vi "Begin.vi"(8 "error in":errorcluster) -> (0 "error out":errorcluster)   [LabVIEW 2020]
doc: "Called before other user functions, this VI is expected to open initial I/O refnums, load in file data, and do all program initialization. Notice that the <B>error out</B> terminal is simply used for data flow. Wiring it to other structures or subVIs ensures that this VI runs first."
uses:
  <vilib>/Rock Robotics/WPI/DriverStation/WPI_DriverStationRobotMode2.ctl
  <vilib>/Rock Robotics/WPI/ThirdParty/Phoenix-LabVIEW/Motor Controller/Controls/CTRE_Phoenix_MotorControl_FeedbackDevice_TalonFX.ctl
  <vilib>/Rock Robotics/WPI/ThirdParty/Phoenix-LabVIEW/Motor Controller/Controls/CTRE_Phoenix_MotorControl_SupplyCurrentLimitConfiguration.ctl
  <vilib>/Rock Robotics/WPI/ThirdParty/Phoenix-LabVIEW/Motor Controller/Controls/CTRE_Phoenix_MotorControl_ControlMode.ctl
  <vilib>/Rock Robotics/WPI/ThirdParty/Phoenix-LabVIEW/Motor Controller/Controls/CTRE_Phoenix_MotorControl_NeutralMode.ctl
  <vilib>/Rock Robotics/WPI/Joystick/WPI_JoystickDeviceEnum.ctl
  <vilib>/Rock Robotics/WPI/ThirdParty/Phoenix-LabVIEW/CANCoder/Controls/CTRE_Phoenix_CANcoder_AbsoluteSensorRange.ctl
  Robot Global Data.vi
  <vilib>/Rock Robotics/Network Tables/NT Write Number.vi
  <vilib>/Rock Robotics/WPI/ThirdParty/Phoenix-LabVIEW/Motor Controller/Sensor/CTRE_Phoenix_MotorControl_SetIntegratedSensorPosition_TalonFX.vi
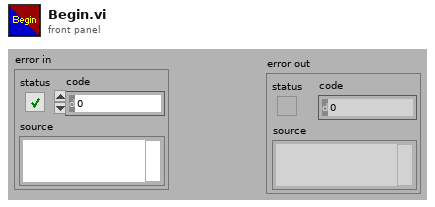
[diagram p1: front panel]
types:
  T1 = typedef "CTRE_Phoenix_CANcoder_AbsoluteSensorRange.ctl" = enum16{"Unsigned [0 to 360)", "Signed [-180 to +180)"}
  T2 = typedef "WPI_JoystickDeviceEnum.ctl" = enum16{"USB 0", "USB 1", "USB 2", "USB 3", "USB 4", "USB 5"}
  T3 = typedef "CTRE_Phoenix_MotorControl_SupplyCurrentLimitConfiguration.ctl" = cluster{"Enable?":bool, "Current Limit":dbl, "Threshold Current":dbl, "Threshold Time":dbl}
  T4 = typedef "CTRE_Phoenix_MotorControl_NeutralMode.ctl" = enum8{"EEPROMSetting", "Override to Coast", "Override to Brake"}
  T5 = typedef "CTRE_Phoenix_MotorControl_ControlMode.ctl" = u16
  T6 = typedef "CTRE_Phoenix_MotorControl_FeedbackDevice_TalonFX.ctl" = i8
  T7 = typedef "WPI_DriverStationRobotMode2.ctl" = enum16{"Autonomous Disabled", "Autonomous Enabled", "Teleop Disabled", "Teleop Enabled", "Disconnected", "Finish", "Test Disabled", "Test Enabled", "Emergency Stopped"}
  T8 = typedef "CTRE_Phoenix_CANcoder_DeviceRef.ctl" = cluster{"DeviceStatus":errorcluster, "Device Number":u8, "Handle":u64, "UsageFrame":u32, "Library Path":path}
  T9 = typedef "WPI_JoystickDevRef.ctl" = cluster{"Device":T2}
  T10 = typedef "WPI_MotorControlDeviceRef.ctl" = cluster{"DeviceStatus":errorcluster, "Type":T11, "PWM":cluster{"PWM Channel":T12, "DeadBand":T13}, "CAN":cluster{"Device Number":u8, "SetOutput VI Ref":variant, "GetOutput VI Ref":variant, "Enable VI Ref":variant, "Disable VI Ref":variant, "Data":variant}, "Invert":bool, "DIO PWM":cluster{"PWM \"Enable\" Channel":T12, "DIOChannel":T14, "PWM Rate":dbl}}
  T11 = typedef "WPI_MotorControlType.ctl" = enum16{"PWM", "CAN", "DIO PWM"}
  T12 = typedef "FPGA_DIOPWMChannel.ctl" = enum8{"PWM 0", "PWM 1", "PWM 2", "PWM 3", "PWM 4", "PWM 5", "PWM 6", "PWM 7", "PWM 8", "PWM 9", "PWM MXP 0", "PWM MXP 1", "PWM MXP 2", "PWM MXP 3", "PWM MXP 4", "PWM MXP 5", "PWM MXP 6", "PWM MXP 7", "PWM MXP 8", "PWM MXP 9", "Invalid"}
  T13 = typedef "WPI_PWMDeadband.ctl" = cluster{"Name":string, "maxPositivePwm":i32, "minPositivePwm":i32, "centerPwm":i32, "maxNegativePwm":i32, "minNegativePwm":i32, "angularRange":u16}
  T14 = typedef "FPGA_DIOChannel.ctl" = enum8{"DIO 0", "DIO 1", "DIO 2", "DIO 3", "DIO 4", "DIO 5", "DIO 6", "DIO 7", "DIO 8", "DIO 9", "DIO MXP 0", "DIO MXP 1", "DIO MXP 2", "DIO MXP 3", "DIO MXP 4", "DIO MXP 5", "DIO MXP 6", "DIO MXP 7", "DIO MXP 8", "DIO MXP 9", "DIO MXP 10", "DIO MXP 11", "DIO MXP 12", "DIO MXP 13", "DIO MXP 14", "DIO MXP 15", "SPI Port CS1", "SPI Port CS2", "SPI Port CS3", "SPI Port MISO", "SPI Port MOSI", "Invalid"}
  T15 = typedef "CTRE_PigeonIMU_DeviceRef.ctl" = cluster{"DeviceStatus":errorcluster, "Device Number":u8, "Type":T16, "Device ID":u32, "Handle":u64, "UsageFrame":u32, "Library Path":path}
  T16 = typedef "CTRE_PigeonIMU_ConnectionType.ctl" = u32
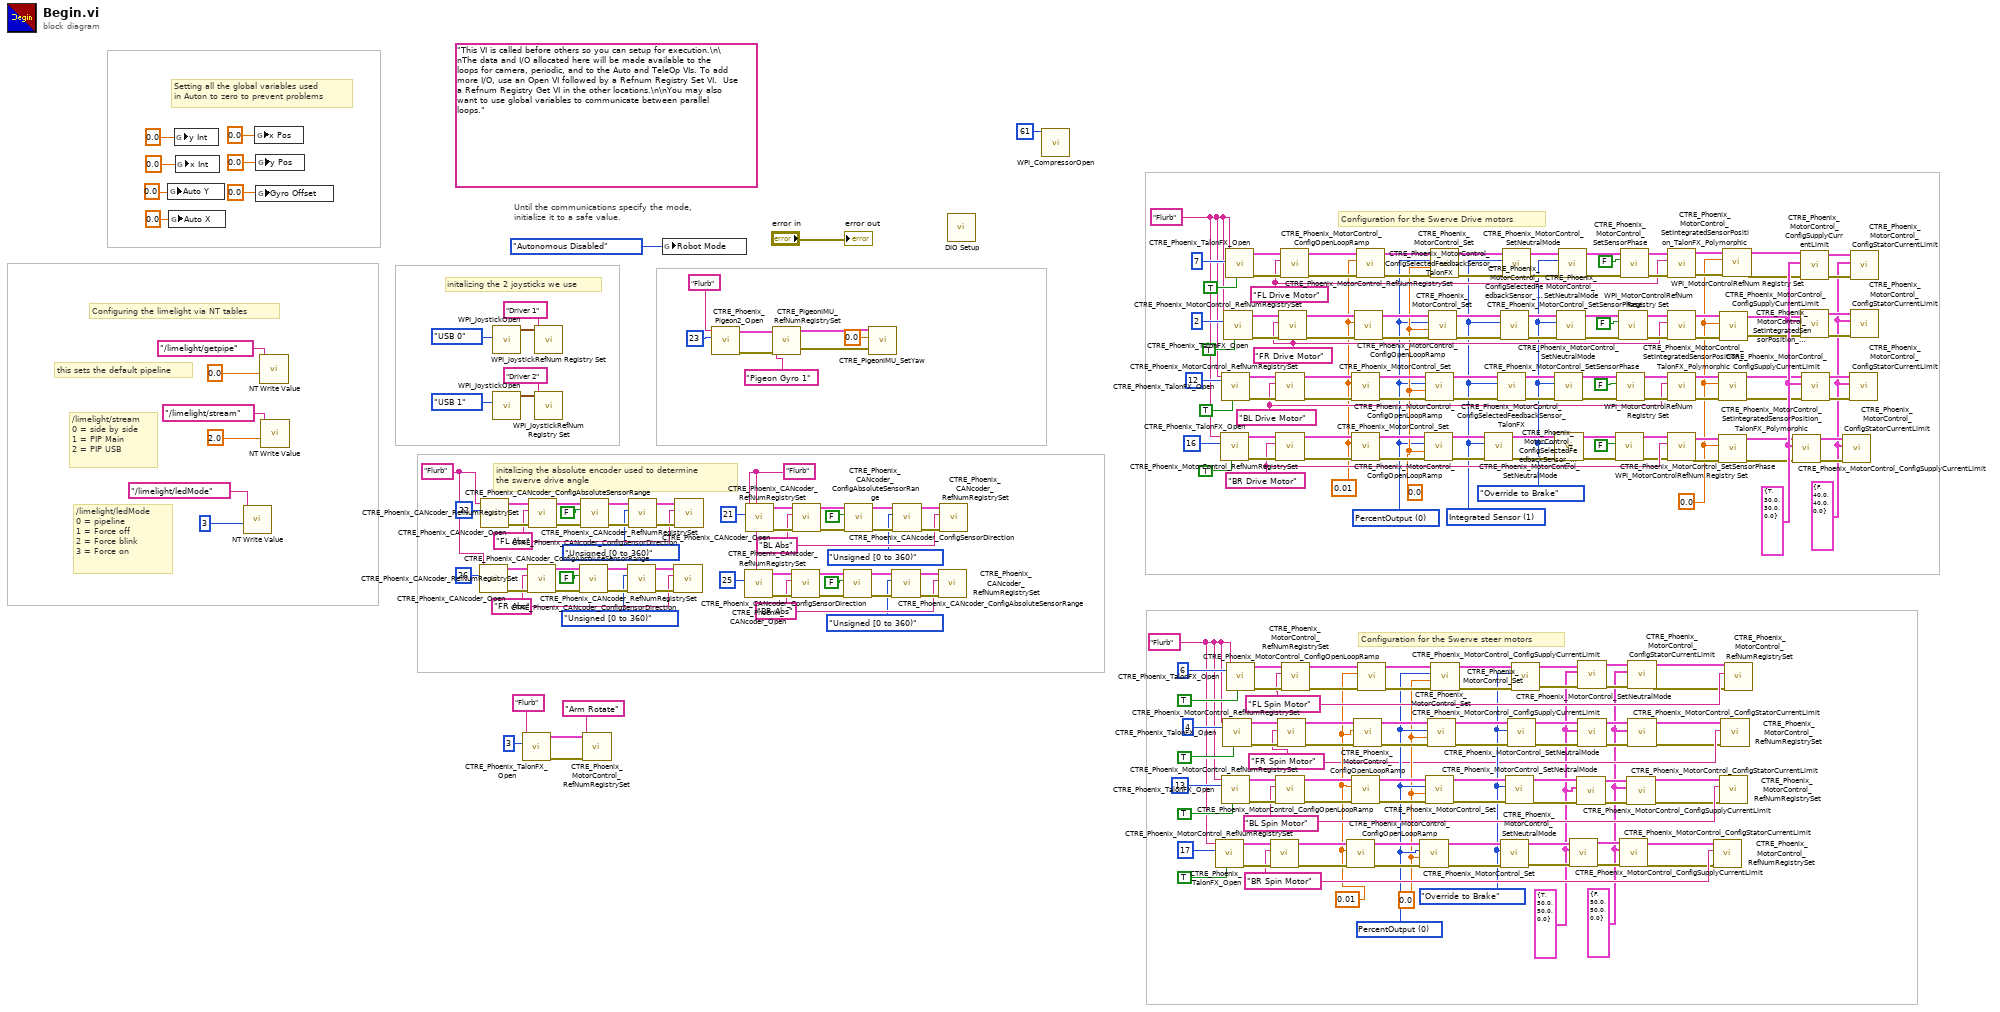
[diagram p0: block diagram]
diagram:
  w7 = "Flurb" ("CAN Bus")
  w8 = "Flurb" ("CAN Bus")
  w9 = "Flurb" ("CAN Bus")
  w10 = "Flurb" ("CAN Bus")
  w14 = "BR Abs" ("refnum name")
  w26 = "BL Abs" ("refnum name")
  w38 = "FR Abs" ("refnum name")
  w50 = "FL Abs" ("refnum name")
  w86 = T3 {"Enable?"=FALSE, "Current Limit"=50.0, "Threshold Current"=50.0, "Threshold Time"=0.0} ("Supply Current Limit Configuration")
  w87 = T3 {"Enable?"=TRUE, "Current Limit"=50.0, "Threshold Current"=50.0, "Threshold Time"=0.0} ("Supply Current Limit Configuration")
  w116 = CTRE_Phoenix_MotorControl_NeutralMode."Override to Brake" ("Motor Control Neutral Mode")
  w114 = 0.0 ("Output")
  w115 = T5 0 items=["PercentOutput"=0, "Position"=1, "Velocity"=2, "Current"=3, "Follower"=5, "MotionProfile"=6, "MotionMagic"=7, "MotionProfileArc"=10, "Disabled"=15] ("Control Mode")
  w113 = 0.01 ("secondsFromNeutralToFull")
  w117 = "BR Spin Motor" ("refnum name")
  w118 = "BL Spin Motor" ("refnum name")
  w110 = "FR Spin Motor" ("refnum name")
  w119 = "FL Spin Motor" ("refnum name")
  w161 = T3 {"Enable?"=FALSE, "Current Limit"=40.0, "Threshold Current"=40.0, "Threshold Time"=0.0} ("Supply Current Limit Configuration")
  w170 = T3 {"Enable?"=TRUE, "Current Limit"=30.0, "Threshold Current"=30.0, "Threshold Time"=0.0} ("Supply Current Limit Configuration")
  w160 = 0.0 ("New Position")
  w187 = CTRE_Phoenix_MotorControl_NeutralMode."Override to Brake" ("Motor Control Neutral Mode")
  w188 = T6 1 items=["Integrated Sensor"=1, "Sensor Sum (S0 + S1)"=9, "Sensor Difference (D0 - D1)"=10, "Remote Source 0"=11, "Remote Source 1"=12, "None"=14, "Software Emulated"=15] ("Talon FX Feedback Device")
  w190 = 0.0 ("Output")
  w189 = T5 0 items=["PercentOutput"=0, "Position"=1, "Velocity"=2, "Current"=3, "Follower"=5, "MotionProfile"=6, "MotionMagic"=7, "MotionProfileArc"=10, "Disabled"=15] ("Control Mode")
  w191 = 0.01 ("secondsFromNeutralToFull")
  w247 = "BR Drive Motor" ("refnum name")
  w192 = "BL Drive Motor" ("refnum name")
  w210 = "FR Drive Motor" ("refnum name")
  w229 = "FL Drive Motor" ("refnum name")
  (unwired) "This VI is called before others so you can setup for execution.\n\nThe data and I/O allocated here will be made available to the loops for camera, periodic, and to the Auto and TeleOp VIs. To add more I/O, use an Open VI followed by a Refnum Registry Set VI.  Use a Refnum Registry Get VI in the other locations.\n\nYou may also want to use global variables to communicate between parallel loops."
  # "initalizing the absolute encoder used to determine\nthe swerve drive angle"
  # "Setting all the global variables used \nin Auton to zero to prevent problems"
  # "Configuring the limelight via NT tables"
  # "initalizing the 2 joysticks we use"
  # "/limelight/ledMode\n0 = pipeline\n1 = Force off\n2 = Force blink\n3 = Force on"
  # "this sets the default pipeline"
  # "/limelight/stream\n0 = side by side\n1 = PIP Main\n2 = PIP USB"
  # "Configuration for the Swerve steer motors"
  # "Configuration for the Swerve Drive motors"
  # "Until the communications specify the mode,\ninitialize it to a safe value."
  n1 = global write "Robot Global Data.vi" "Auto Y"(0.0 ("Auto Y")) -> ()
  n2 = global write "Robot Global Data.vi" "Auto X"(0.0 ("Auto Y")) -> ()
  n3 = global write "Robot Global Data.vi" "y Int"(0.0 ("Auto Y")) -> ()
  n4 = global write "Robot Global Data.vi" "x Int"(0.0 ("Auto Y")) -> ()
  n5 = call-poly <vilib>:"NT Write Value.vi"("value"=3, "name"="/limelight/ledMode" ("Name")) -> ()  [unwired: 9 in, 1 out]
  n6 = global write "Robot Global Data.vi" "x Pos"(0.0 ("Auto Y")) -> ()
  n7 = global write "Robot Global Data.vi" "y Pos"(0.0 ("Auto Y")) -> ()
  n8 = global write "Robot Global Data.vi" "Gyro Offset"(0.0 ("Auto Y")) -> ()
  n9 = call-poly <vilib>:"NT Write Value.vi"("value"=0.0 ("Numeric"), "name"="/limelight/getpipe" ("Name")) -> ()  [unwired: 9 in, 1 out]
  n10 = call-poly <vilib>:"NT Write Value.vi"("value"=2.0 ("Numeric"), "name"="/limelight/stream" ("Name")) -> ()  [unwired: 9 in, 1 out]
  n11 = call <vilib>:"CTRE_Phoenix_CANcoder_Open.vi"("Device Number"=u8 26, "CAN Bus"=w8) -> ("error out"=w47:errorcluster, "CTRE_CANcoder_DeviceRef"=w46:T8)  [unwired: 8 in]
  n12 = call <vilib>:"CTRE_Phoenix_CANcoder_Open.vi"("Device Number"=u8 22, "CAN Bus"=w8) -> ("error out"=w59:errorcluster, "CTRE_CANcoder_DeviceRef"=w58:T8)  [unwired: 8 in]
  n13 = call <vilib>:"WPI_JoystickOpen.vi"("JoystickDevice"=WPI_JoystickDeviceEnum."USB 0") -> ("JoystickDevRef"=w85:T9)  [unwired: 10 in]
  n14 = call <vilib>:"WPI_JoystickOpen.vi"("JoystickDevice"=WPI_JoystickDeviceEnum."USB 1") -> ("JoystickDevRef"=w75:T9)  [unwired: 10 in]
  n15 = call <vilib>:"CTRE_Phoenix_TalonFX_Open.vi"("Device Number"=u8 3, "CAN Bus"="Flurb") -> ("error out"=w6:errorcluster, "PhoenixMotorControlDevRef"=w5:T10)  [unwired: 8 in]
  n16 = call <vilib>:"CTRE_Phoenix_CANcoder_RefNumRegistrySet.vi"("error in (no error)"=w47, "refnum name"=w38, "CTRE_CANcoder_DeviceRef"=w46) -> ("error out"=w45:errorcluster, "CTRE_CANcoder_DeviceRef"=w44:T8)  [unwired: 7 in]
  n17 = call <vilib>:"CTRE_Phoenix_CANcoder_RefNumRegistrySet.vi"("error in (no error)"=w59, "refnum name"=w50, "CTRE_CANcoder_DeviceRef"=w58) -> ("error out"=w57:errorcluster, "CTRE_CANcoder_DeviceRef"=w56:T8)  [unwired: 7 in]
  n18 = call <vilib>:"WPI_JoystickRefNum Registry Set.vi"("refnum name"="Driver 1", "JoystickDevRef"=w85) -> ()  [unwired: 8 in, 2 out]
  n19 = call <vilib>:"WPI_JoystickRefNum Registry Set.vi"("refnum name"="Driver 2", "JoystickDevRef"=w75) -> ()  [unwired: 8 in, 2 out]
  n20 = call <vilib>:"CTRE_Phoenix_CANcoder_ConfigSensorDirection.vi"("error in"=w45, "Sensor Direction"=FALSE, "CTRE_CANcoder_DeviceRef"=w44) -> ("error out"=w43:errorcluster, "CTRE_CANcoder_DeviceRef"=w42:T8)  [unwired: 7 in]
  n21 = call <vilib>:"CTRE_Phoenix_CANcoder_ConfigSensorDirection.vi"("error in"=w57, "Sensor Direction"=FALSE, "CTRE_CANcoder_DeviceRef"=w56) -> ("error out"=w55:errorcluster, "CTRE_CANcoder_DeviceRef"=w54:T8)  [unwired: 7 in]
  n22 = call <vilib>:"CTRE_Phoenix_MotorControl_RefNumRegistrySet.vi"("error in (no error)"=w6, "refnum name"="Arm Rotate", "PhoenixMotorControlDevRef"=w5) -> ()  [unwired: 7 in, 2 out]
  n23 = call <vilib>:"CTRE_Phoenix_CANcoder_ConfigAbsoluteSensorRange.vi"("error in"=w43, "Absolute Sensor Range"=CTRE_Phoenix_CANcoder_AbsoluteSensorRange."Unsigned [0 to 360)", "CTRE_CANcoder_DeviceRef"=w42) -> ("error out"=w41:errorcluster, "CTRE_CANcoder_DeviceRef"=w40:T8)  [unwired: 7 in]
  n24 = call <vilib>:"CTRE_Phoenix_CANcoder_ConfigAbsoluteSensorRange.vi"("error in"=w55, "Absolute Sensor Range"=CTRE_Phoenix_CANcoder_AbsoluteSensorRange."Unsigned [0 to 360)", "CTRE_CANcoder_DeviceRef"=w54) -> ("error out"=w53:errorcluster, "CTRE_CANcoder_DeviceRef"=w52:T8)  [unwired: 7 in]
  n25 = global write "Robot Global Data.vi" "Robot Mode"(WPI_DriverStationRobotMode2."Autonomous Disabled" ("Robot Mode")) -> ()
  n26 = call <vilib>:"CTRE_Phoenix_CANcoder_RefNumRegistrySet.vi"("error in (no error)"=w41, "refnum name"=w38, "CTRE_CANcoder_DeviceRef"=w40) -> ()  [unwired: 7 in, 2 out]
  n27 = call <vilib>:"CTRE_Phoenix_CANcoder_RefNumRegistrySet.vi"("error in (no error)"=w53, "refnum name"=w50, "CTRE_CANcoder_DeviceRef"=w52) -> ()  [unwired: 7 in, 2 out]
  n28 = call <vilib>:"CTRE_Phoenix_Pigeon2_Open.vi"("Device Number"=u8 23, "canbus"="Flurb") -> ("error out"=w82:errorcluster, "PigeonIMUDevRef"=w81:T15)  [unwired: 8 in]
  n29 = call <vilib>:"CTRE_Phoenix_CANcoder_Open.vi"("Device Number"=u8 25, "CAN Bus"=w7) -> ("error out"=w23:errorcluster, "CTRE_CANcoder_DeviceRef"=w22:T8)  [unwired: 8 in]
  n30 = call <vilib>:"CTRE_Phoenix_CANcoder_Open.vi"("Device Number"=u8 21, "CAN Bus"=w7) -> ("error out"=w35:errorcluster, "CTRE_CANcoder_DeviceRef"=w34:T8)  [unwired: 8 in]
  n31 = call <vilib>:"CTRE_PigeonIMU_RefNumRegistrySet.vi"("error in (no error)"=w82, "refnum name"="Pigeon Gyro 1", "PigeonIMUDevRef"=w81) -> ("error out"=w77:errorcluster, "PigeonIMUDevRef"=w78:T15)  [unwired: 7 in]
  n32 = call <vilib>:"CTRE_Phoenix_CANcoder_RefNumRegistrySet.vi"("error in (no error)"=w23, "refnum name"=w14, "CTRE_CANcoder_DeviceRef"=w22) -> ("error out"=w21:errorcluster, "CTRE_CANcoder_DeviceRef"=w20:T8)  [unwired: 7 in]
  n33 = call <vilib>:"CTRE_Phoenix_CANcoder_RefNumRegistrySet.vi"("error in (no error)"=w35, "refnum name"=w26, "CTRE_CANcoder_DeviceRef"=w34) -> ("error out"=w33:errorcluster, "CTRE_CANcoder_DeviceRef"=w32:T8)  [unwired: 7 in]
  n34 = call <vilib>:"CTRE_Phoenix_CANcoder_ConfigSensorDirection.vi"("error in"=w21, "Sensor Direction"=FALSE, "CTRE_CANcoder_DeviceRef"=w20) -> ("error out"=w19:errorcluster, "CTRE_CANcoder_DeviceRef"=w18:T8)  [unwired: 7 in]
  n35 = call <vilib>:"CTRE_Phoenix_CANcoder_ConfigSensorDirection.vi"("error in"=w33, "Sensor Direction"=FALSE, "CTRE_CANcoder_DeviceRef"=w32) -> ("error out"=w31:errorcluster, "CTRE_CANcoder_DeviceRef"=w30:T8)  [unwired: 7 in]
  n36 = call <vilib>:"CTRE_PigeonIMU_SetYaw.vi"("error in (no error)"=w77, "Value"=0.0, "PigeonIMUDevRef"=w78) -> ()  [unwired: 7 in, 2 out]
  n37 = call <vilib>:"CTRE_Phoenix_CANcoder_ConfigAbsoluteSensorRange.vi"("error in"=w19, "Absolute Sensor Range"=CTRE_Phoenix_CANcoder_AbsoluteSensorRange."Unsigned [0 to 360)", "CTRE_CANcoder_DeviceRef"=w18) -> ("error out"=w17:errorcluster, "CTRE_CANcoder_DeviceRef"=w16:T8)  [unwired: 7 in]
  n38 = call <vilib>:"CTRE_Phoenix_CANcoder_ConfigAbsoluteSensorRange.vi"("error in"=w31, "Absolute Sensor Range"=CTRE_Phoenix_CANcoder_AbsoluteSensorRange."Unsigned [0 to 360)", "CTRE_CANcoder_DeviceRef"=w30) -> ("error out"=w29:errorcluster, "CTRE_CANcoder_DeviceRef"=w28:T8)  [unwired: 7 in]
  n39 = call <vilib>:"CTRE_Phoenix_CANcoder_RefNumRegistrySet.vi"("error in (no error)"=w17, "refnum name"=w14, "CTRE_CANcoder_DeviceRef"=w16) -> ()  [unwired: 7 in, 2 out]
  n40 = call <vilib>:"CTRE_Phoenix_CANcoder_RefNumRegistrySet.vi"("error in (no error)"=w29, "refnum name"=w26, "CTRE_CANcoder_DeviceRef"=w28) -> ()  [unwired: 7 in, 2 out]
  n41 = call "DIO Setup.vi"() -> ()  [unwired: 12 in]
  n42 = call <vilib>:"WPI_CompressorOpen.vi"("Pneumatics device (def)"=u8 61) -> ()  [unwired: 13 in, 2 out]
  n43 = call <vilib>:"CTRE_Phoenix_TalonFX_Open.vi"("Invert"=TRUE, "Device Number"=u8 17, "CAN Bus"=w9) -> ("error out"=w132:errorcluster, "PhoenixMotorControlDevRef"=w131:T10)  [unwired: 7 in]
  n44 = call <vilib>:"CTRE_Phoenix_TalonFX_Open.vi"("Invert"=TRUE, "Device Number"=u8 16, "CAN Bus"=w10) -> ("error out"=w263:errorcluster, "PhoenixMotorControlDevRef"=w262:T10)  [unwired: 7 in]
  n45 = call <vilib>:"CTRE_Phoenix_TalonFX_Open.vi"("Invert"=TRUE, "Device Number"=u8 12, "CAN Bus"=w10) -> ("error out"=w209:errorcluster, "PhoenixMotorControlDevRef"=w208:T10)  [unwired: 7 in]
  n46 = call <vilib>:"CTRE_Phoenix_TalonFX_Open.vi"("Invert"=TRUE, "Device Number"=u8 13, "CAN Bus"=w9) -> ("error out"=w141:errorcluster, "PhoenixMotorControlDevRef"=w140:T10)  [unwired: 7 in]
  n47 = call <vilib>:"CTRE_Phoenix_TalonFX_Open.vi"("Invert"=TRUE, "Device Number"=u8 4, "CAN Bus"=w9) -> ("error out"=w150:errorcluster, "PhoenixMotorControlDevRef"=w149:T10)  [unwired: 7 in]
  n48 = call <vilib>:"CTRE_Phoenix_TalonFX_Open.vi"("Invert"=TRUE, "Device Number"=u8 2, "CAN Bus"=w10) -> ("error out"=w227:errorcluster, "PhoenixMotorControlDevRef"=w226:T10)  [unwired: 7 in]
  n49 = call <vilib>:"CTRE_Phoenix_TalonFX_Open.vi"("Invert"=TRUE, "Device Number"=u8 7, "CAN Bus"=w10) -> ("error out"=w245:errorcluster, "PhoenixMotorControlDevRef"=w244:T10)  [unwired: 7 in]
  n50 = call <vilib>:"CTRE_Phoenix_TalonFX_Open.vi"("Invert"=TRUE, "Device Number"=u8 6, "CAN Bus"=w9) -> ("error out"=w159:errorcluster, "PhoenixMotorControlDevRef"=w158:T10)  [unwired: 7 in]
  n51 = call <vilib>:"CTRE_Phoenix_MotorControl_RefNumRegistrySet.vi"("error in (no error)"=w132, "refnum name"=w117, "PhoenixMotorControlDevRef"=w131) -> ("error out"=w129:errorcluster, "PhoenixMotorControlDevRef"=w130:T10)  [unwired: 7 in]
  n52 = call <vilib>:"CTRE_Phoenix_MotorControl_RefNumRegistrySet.vi"("error in (no error)"=w209, "refnum name"=w192, "PhoenixMotorControlDevRef"=w208) -> ("error out"=w206:errorcluster, "PhoenixMotorControlDevRef"=w207:T10)  [unwired: 7 in]
  n53 = call <vilib>:"CTRE_Phoenix_MotorControl_RefNumRegistrySet.vi"("error in (no error)"=w263, "refnum name"=w247, "PhoenixMotorControlDevRef"=w262) -> ("error out"=w260:errorcluster, "PhoenixMotorControlDevRef"=w261:T10)  [unwired: 7 in]
  n54 = call <vilib>:"CTRE_Phoenix_MotorControl_RefNumRegistrySet.vi"("error in (no error)"=w141, "refnum name"=w118, "PhoenixMotorControlDevRef"=w140) -> ("error out"=w138:errorcluster, "PhoenixMotorControlDevRef"=w139:T10)  [unwired: 7 in]
  n55 = call <vilib>:"CTRE_Phoenix_MotorControl_RefNumRegistrySet.vi"("error in (no error)"=w150, "refnum name"=w110, "PhoenixMotorControlDevRef"=w149) -> ("error out"=w147:errorcluster, "PhoenixMotorControlDevRef"=w148:T10)  [unwired: 7 in]
  n56 = call <vilib>:"CTRE_Phoenix_MotorControl_RefNumRegistrySet.vi"("error in (no error)"=w227, "refnum name"=w210, "PhoenixMotorControlDevRef"=w226) -> ("error out"=w224:errorcluster, "PhoenixMotorControlDevRef"=w225:T10)  [unwired: 7 in]
  n57 = call <vilib>:"CTRE_Phoenix_MotorControl_RefNumRegistrySet.vi"("error in (no error)"=w245, "refnum name"=w229, "PhoenixMotorControlDevRef"=w244) -> ("error out"=w242:errorcluster, "PhoenixMotorControlDevRef"=w243:T10)  [unwired: 7 in]
  n58 = call <vilib>:"CTRE_Phoenix_MotorControl_RefNumRegistrySet.vi"("error in (no error)"=w159, "refnum name"=w119, "PhoenixMotorControlDevRef"=w158) -> ("error out"=w156:errorcluster, "PhoenixMotorControlDevRef"=w157:T10)  [unwired: 7 in]
  n59 = call <vilib>:"CTRE_Phoenix_MotorControl_ConfigOpenLoopRamp.vi"("error in (no error)"=w129, "secondsFromNeutralToFull"=w113, "PhoenixMotorControlDevRef"=w130) -> ("error out"=w128:errorcluster, "PhoenixMotorControlDevRef"=w127:T10)  [unwired: 7 in]
  n60 = call <vilib>:"CTRE_Phoenix_MotorControl_ConfigOpenLoopRamp.vi"("error in (no error)"=w206, "secondsFromNeutralToFull"=w191, "PhoenixMotorControlDevRef"=w207) -> ("error out"=w205:errorcluster, "PhoenixMotorControlDevRef"=w204:T10)  [unwired: 7 in]
  n61 = call <vilib>:"CTRE_Phoenix_MotorControl_ConfigOpenLoopRamp.vi"("error in (no error)"=w260, "secondsFromNeutralToFull"=w191, "PhoenixMotorControlDevRef"=w261) -> ("error out"=w259:errorcluster, "PhoenixMotorControlDevRef"=w258:T10)  [unwired: 7 in]
  n62 = call <vilib>:"CTRE_Phoenix_MotorControl_ConfigOpenLoopRamp.vi"("error in (no error)"=w138, "secondsFromNeutralToFull"=w113, "PhoenixMotorControlDevRef"=w139) -> ("error out"=w137:errorcluster, "PhoenixMotorControlDevRef"=w136:T10)  [unwired: 7 in]
  n63 = call <vilib>:"CTRE_Phoenix_MotorControl_ConfigOpenLoopRamp.vi"("error in (no error)"=w147, "secondsFromNeutralToFull"=w113, "PhoenixMotorControlDevRef"=w148) -> ("error out"=w146:errorcluster, "PhoenixMotorControlDevRef"=w145:T10)  [unwired: 7 in]
  n64 = call <vilib>:"CTRE_Phoenix_MotorControl_ConfigOpenLoopRamp.vi"("error in (no error)"=w224, "secondsFromNeutralToFull"=w191, "PhoenixMotorControlDevRef"=w225) -> ("error out"=w223:errorcluster, "PhoenixMotorControlDevRef"=w222:T10)  [unwired: 7 in]
  n65 = call <vilib>:"CTRE_Phoenix_MotorControl_ConfigOpenLoopRamp.vi"("error in (no error)"=w242, "secondsFromNeutralToFull"=w191, "PhoenixMotorControlDevRef"=w243) -> ("error out"=w241:errorcluster, "PhoenixMotorControlDevRef"=w240:T10)  [unwired: 7 in]
  n66 = call <vilib>:"CTRE_Phoenix_MotorControl_ConfigOpenLoopRamp.vi"("error in (no error)"=w156, "secondsFromNeutralToFull"=w113, "PhoenixMotorControlDevRef"=w157) -> ("error out"=w155:errorcluster, "PhoenixMotorControlDevRef"=w154:T10)  [unwired: 7 in]
  n67 = call <vilib>:"CTRE_Phoenix_MotorControl_Set.vi"("error in (no error)"=w128, "Output"=w114, "Control Mode"=w115, "PhoenixMotorControlDevRef"=w127) -> ("error out"=w125:errorcluster, "PhoenixMotorControlDevRef"=w124:T10)  [unwired: 6 in]
  n68 = call <vilib>:"CTRE_Phoenix_MotorControl_Set.vi"("error in (no error)"=w259, "Output"=w190, "Control Mode"=w189, "PhoenixMotorControlDevRef"=w258) -> ("error out"=w257:errorcluster, "PhoenixMotorControlDevRef"=w256:T10)  [unwired: 6 in]
  n69 = call <vilib>:"CTRE_Phoenix_MotorControl_Set.vi"("error in (no error)"=w205, "Output"=w190, "Control Mode"=w189, "PhoenixMotorControlDevRef"=w204) -> ("error out"=w203:errorcluster, "PhoenixMotorControlDevRef"=w202:T10)  [unwired: 6 in]
  n70 = call <vilib>:"CTRE_Phoenix_MotorControl_Set.vi"("error in (no error)"=w137, "Output"=w114, "Control Mode"=w115, "PhoenixMotorControlDevRef"=w136) -> ("error out"=w134:errorcluster, "PhoenixMotorControlDevRef"=w133:T10)  [unwired: 6 in]
  n71 = call <vilib>:"CTRE_Phoenix_MotorControl_Set.vi"("error in (no error)"=w146, "Output"=w114, "Control Mode"=w115, "PhoenixMotorControlDevRef"=w145) -> ("error out"=w143:errorcluster, "PhoenixMotorControlDevRef"=w142:T10)  [unwired: 6 in]
  n72 = call <vilib>:"CTRE_Phoenix_MotorControl_Set.vi"("error in (no error)"=w223, "Output"=w190, "Control Mode"=w189, "PhoenixMotorControlDevRef"=w222) -> ("error out"=w221:errorcluster, "PhoenixMotorControlDevRef"=w220:T10)  [unwired: 6 in]
  n73 = call <vilib>:"CTRE_Phoenix_MotorControl_Set.vi"("error in (no error)"=w241, "Output"=w190, "Control Mode"=w189, "PhoenixMotorControlDevRef"=w240) -> ("error out"=w239:errorcluster, "PhoenixMotorControlDevRef"=w238:T10)  [unwired: 6 in]
  n74 = call <vilib>:"CTRE_Phoenix_MotorControl_Set.vi"("error in (no error)"=w155, "Output"=w114, "Control Mode"=w115, "PhoenixMotorControlDevRef"=w154) -> ("error out"=w152:errorcluster, "PhoenixMotorControlDevRef"=w151:T10)  [unwired: 6 in]
  n75 = call <vilib>:"CTRE_Phoenix_MotorControl_ConfigSelectedFeedbackSensor_TalonFX.vi"("error in (no error)"=w257, "Talon FX Feedback Device"=w188, "PhoenixMotorControlDevRef"=w256) -> ("error out"=w255:errorcluster, "PhoenixMotorControlDevRef"=w254:T10)  [unwired: 7 in]
  n76 = call <vilib>:"CTRE_Phoenix_MotorControl_ConfigSelectedFeedbackSensor_TalonFX.vi"("error in (no error)"=w203, "Talon FX Feedback Device"=w188, "PhoenixMotorControlDevRef"=w202) -> ("error out"=w201:errorcluster, "PhoenixMotorControlDevRef"=w200:T10)  [unwired: 7 in]
  n77 = call <vilib>:"CTRE_Phoenix_MotorControl_ConfigSelectedFeedbackSensor_TalonFX.vi"("error in (no error)"=w221, "Talon FX Feedback Device"=w188, "PhoenixMotorControlDevRef"=w220) -> ("error out"=w219:errorcluster, "PhoenixMotorControlDevRef"=w218:T10)  [unwired: 7 in]
  n78 = call <vilib>:"CTRE_Phoenix_MotorControl_SetNeutralMode.vi"("error in (no error)"=w125, "Motor Control Neutral Mode"=w116, "PhoenixMotorControlDevRef"=w124) -> ("error out"=w96:errorcluster, "PhoenixMotorControlDevRef"=w97:T10)  [unwired: 7 in]
  n79 = call <vilib>:"CTRE_Phoenix_MotorControl_ConfigSelectedFeedbackSensor_TalonFX.vi"("error in (no error)"=w239, "Talon FX Feedback Device"=w188, "PhoenixMotorControlDevRef"=w238) -> ("error out"=w237:errorcluster, "PhoenixMotorControlDevRef"=w236:T10)  [unwired: 7 in]
  n80 = call <vilib>:"CTRE_Phoenix_MotorControl_SetNeutralMode.vi"("error in (no error)"=w134, "Motor Control Neutral Mode"=w116, "PhoenixMotorControlDevRef"=w133) -> ("error out"=w98:errorcluster, "PhoenixMotorControlDevRef"=w99:T10)  [unwired: 7 in]
  n81 = call <vilib>:"CTRE_Phoenix_MotorControl_SetNeutralMode.vi"("error in (no error)"=w143, "Motor Control Neutral Mode"=w116, "PhoenixMotorControlDevRef"=w142) -> ("error out"=w101:errorcluster, "PhoenixMotorControlDevRef"=w100:T10)  [unwired: 7 in]
  n82 = call <vilib>:"CTRE_Phoenix_MotorControl_SetNeutralMode.vi"("error in (no error)"=w152, "Motor Control Neutral Mode"=w116, "PhoenixMotorControlDevRef"=w151) -> ("error out"=w102:errorcluster, "PhoenixMotorControlDevRef"=w103:T10)  [unwired: 7 in]
  n83 = call <vilib>:"CTRE_Phoenix_MotorControl_SetNeutralMode.vi"("error in (no error)"=w201, "Motor Control Neutral Mode"=w187, "PhoenixMotorControlDevRef"=w200) -> ("error out"=w199:errorcluster, "PhoenixMotorControlDevRef"=w198:T10)  [unwired: 7 in]
  n84 = call <vilib>:"CTRE_Phoenix_MotorControl_SetNeutralMode.vi"("error in (no error)"=w255, "Motor Control Neutral Mode"=w187, "PhoenixMotorControlDevRef"=w254) -> ("error out"=w253:errorcluster, "PhoenixMotorControlDevRef"=w252:T10)  [unwired: 7 in]
  n85 = call <vilib>:"CTRE_Phoenix_MotorControl_SetNeutralMode.vi"("error in (no error)"=w219, "Motor Control Neutral Mode"=w187, "PhoenixMotorControlDevRef"=w218) -> ("error out"=w217:errorcluster, "PhoenixMotorControlDevRef"=w216:T10)  [unwired: 7 in]
  n86 = call <vilib>:"CTRE_Phoenix_MotorControl_SetNeutralMode.vi"("error in (no error)"=w237, "Motor Control Neutral Mode"=w187, "PhoenixMotorControlDevRef"=w236) -> ("error out"=w235:errorcluster, "PhoenixMotorControlDevRef"=w234:T10)  [unwired: 7 in]
  n87 = call <vilib>:"CTRE_Phoenix_MotorControl_ConfigSupplyCurrentLimit.vi"("error in (no error)"=w96, "Supply Current Limit Configuration"=w87, "PhoenixMotorControlDevRef"=w97) -> ("error out"=w105:errorcluster, "PhoenixMotorControlDevRef"=w104:T10)  [unwired: 7 in]
  n88 = call <vilib>:"CTRE_Phoenix_MotorControl_ConfigSupplyCurrentLimit.vi"("error in (no error)"=w98, "Supply Current Limit Configuration"=w87, "PhoenixMotorControlDevRef"=w99) -> ("error out"=w107:errorcluster, "PhoenixMotorControlDevRef"=w106:T10)  [unwired: 7 in]
  n89 = call <vilib>:"CTRE_Phoenix_MotorControl_ConfigSupplyCurrentLimit.vi"("error in (no error)"=w102, "Supply Current Limit Configuration"=w87, "PhoenixMotorControlDevRef"=w103) -> ("error out"=w112:errorcluster, "PhoenixMotorControlDevRef"=w111:T10)  [unwired: 7 in]
  n90 = call <vilib>:"CTRE_Phoenix_MotorControl_ConfigSupplyCurrentLimit.vi"("error in (no error)"=w101, "Supply Current Limit Configuration"=w87, "PhoenixMotorControlDevRef"=w100) -> ("error out"=w109:errorcluster, "PhoenixMotorControlDevRef"=w108:T10)  [unwired: 7 in]
  n91 = call <vilib>:"CTRE_Phoenix_MotorControl_SetSensorPhase.vi"("error in (no error)"=w253, "PhaseSensor"=FALSE, "PhoenixMotorControlDevRef"=w252) -> ("error out"=w246:errorcluster, "PhoenixMotorControlDevRef"=w248:T10)  [unwired: 7 in]
  n92 = call <vilib>:"CTRE_Phoenix_MotorControl_SetSensorPhase.vi"("error in (no error)"=w199, "PhaseSensor"=FALSE, "PhoenixMotorControlDevRef"=w198) -> ("error out"=w194:errorcluster, "PhoenixMotorControlDevRef"=w195:T10)  [unwired: 7 in]
  n93 = call <vilib>:"CTRE_Phoenix_MotorControl_SetSensorPhase.vi"("error in (no error)"=w217, "PhaseSensor"=FALSE, "PhoenixMotorControlDevRef"=w216) -> ("error out"=w212:errorcluster, "PhoenixMotorControlDevRef"=w213:T10)  [unwired: 7 in]
  n94 = call <vilib>:"CTRE_Phoenix_MotorControl_ConfigStatorCurrentLimit.vi"("error in (no error)"=w105, "Stator Current Limit Configuration"=w86, "PhoenixMotorControlDevRef"=w104) -> ("error out"=w88:errorcluster, "PhoenixMotorControlDevRef"=w89:T10)  [unwired: 7 in]
  n95 = call <vilib>:"CTRE_Phoenix_MotorControl_SetSensorPhase.vi"("error in (no error)"=w235, "PhaseSensor"=FALSE, "PhoenixMotorControlDevRef"=w234) -> ("error out"=w230:errorcluster, "PhoenixMotorControlDevRef"=w231:T10)  [unwired: 7 in]
  n96 = call <vilib>:"CTRE_Phoenix_MotorControl_ConfigStatorCurrentLimit.vi"("error in (no error)"=w107, "Stator Current Limit Configuration"=w86, "PhoenixMotorControlDevRef"=w106) -> ("error out"=w90:errorcluster, "PhoenixMotorControlDevRef"=w91:T10)  [unwired: 7 in]
  n97 = call <vilib>:"CTRE_Phoenix_MotorControl_ConfigStatorCurrentLimit.vi"("error in (no error)"=w112, "Stator Current Limit Configuration"=w86, "PhoenixMotorControlDevRef"=w111) -> ("error out"=w94:errorcluster, "PhoenixMotorControlDevRef"=w95:T10)  [unwired: 7 in]
  n98 = call <vilib>:"CTRE_Phoenix_MotorControl_ConfigStatorCurrentLimit.vi"("error in (no error)"=w109, "Stator Current Limit Configuration"=w86, "PhoenixMotorControlDevRef"=w108) -> ("error out"=w92:errorcluster, "PhoenixMotorControlDevRef"=w93:T10)  [unwired: 7 in]
  n99 = call <vilib>:"WPI_MotorControlRefNum Registry Set.vi"("error in (no error)"=w230, "refnum name"=w229, "MotorControlDevRef"=w231) -> ("error out"=w185:errorcluster, "MotorControlDevRef"=w186:T10)  [unwired: 7 in]
  n100 = call <vilib>:"WPI_MotorControlRefNum Registry Set.vi"("error in (no error)"=w212, "refnum name"=w210, "MotorControlDevRef"=w213) -> ("error out"=w183:errorcluster, "MotorControlDevRef"=w184:T10)  [unwired: 7 in]
  n101 = call <vilib>:"WPI_MotorControlRefNum Registry Set.vi"("error in (no error)"=w194, "refnum name"=w192, "MotorControlDevRef"=w195) -> ("error out"=w181:errorcluster, "MotorControlDevRef"=w182:T10)  [unwired: 7 in]
  n102 = call <vilib>:"WPI_MotorControlRefNum Registry Set.vi"("error in (no error)"=w246, "refnum name"=w247, "MotorControlDevRef"=w248) -> ("error out"=w179:errorcluster, "MotorControlDevRef"=w180:T10)  [unwired: 7 in]
  n103 = call <vilib>:"CTRE_Phoenix_MotorControl_RefNumRegistrySet.vi"("error in (no error)"=w88, "refnum name"=w117, "PhoenixMotorControlDevRef"=w89) -> ()  [unwired: 7 in, 2 out]
  n104 = call-poly <vilib>:"CTRE_Phoenix_MotorControl_SetIntegratedSensorPosition_TalonFX_Polymorphic.vi"("error in (no error)"=w181, "New Position"=w160, "PhoenixMotorControlDevRef"=w182) -> ("error out"=w164:errorcluster, "PhoenixMotorControlDevRef"=w165:T10)  [unwired: 7 in]
  n105 = call-poly <vilib>:"CTRE_Phoenix_MotorControl_SetIntegratedSensorPosition_TalonFX_Polymorphic.vi"("error in (no error)"=w179, "New Position"=w160, "PhoenixMotorControlDevRef"=w180) -> ("error out"=w162:errorcluster, "PhoenixMotorControlDevRef"=w163:T10)  [unwired: 7 in]
  n106 = call-poly <vilib>:"CTRE_Phoenix_MotorControl_SetIntegratedSensorPosition_TalonFX_Polymorphic.vi"("error in (no error)"=w183, "New Position"=w160, "PhoenixMotorControlDevRef"=w184) -> ("error out"=w166:errorcluster, "PhoenixMotorControlDevRef"=w167:T10)  [unwired: 7 in]
  n107 = call <vilib>:"CTRE_Phoenix_MotorControl_RefNumRegistrySet.vi"("error in (no error)"=w90, "refnum name"=w118, "PhoenixMotorControlDevRef"=w91) -> ()  [unwired: 7 in, 2 out]
  n108 = call <vilib>:"CTRE_Phoenix_MotorControl_RefNumRegistrySet.vi"("error in (no error)"=w92, "refnum name"=w110, "PhoenixMotorControlDevRef"=w93) -> ()  [unwired: 7 in, 2 out]
  n109 = call-poly <vilib>:"CTRE_Phoenix_MotorControl_SetIntegratedSensorPosition_TalonFX_Polymorphic.vi"("error in (no error)"=w185, "New Position"=w160, "PhoenixMotorControlDevRef"=w186) -> ("error out"=w168:errorcluster, "PhoenixMotorControlDevRef"=w169:T10)  [unwired: 7 in]
  n110 = call <vilib>:"CTRE_Phoenix_MotorControl_RefNumRegistrySet.vi"("error in (no error)"=w94, "refnum name"=w119, "PhoenixMotorControlDevRef"=w95) -> ()  [unwired: 7 in, 2 out]
  n111 = call <vilib>:"CTRE_Phoenix_MotorControl_ConfigSupplyCurrentLimit.vi"("error in (no error)"=w162, "Supply Current Limit Configuration"=w170, "PhoenixMotorControlDevRef"=w163) -> ("error out"=w172:errorcluster, "PhoenixMotorControlDevRef"=w171:T10)  [unwired: 7 in]
  n112 = call <vilib>:"CTRE_Phoenix_MotorControl_ConfigSupplyCurrentLimit.vi"("error in (no error)"=w168, "Supply Current Limit Configuration"=w170, "PhoenixMotorControlDevRef"=w169) -> ("error out"=w178:errorcluster, "PhoenixMotorControlDevRef"=w177:T10)  [unwired: 7 in]
  n113 = call <vilib>:"CTRE_Phoenix_MotorControl_ConfigSupplyCurrentLimit.vi"("error in (no error)"=w166, "Supply Current Limit Configuration"=w170, "PhoenixMotorControlDevRef"=w167) -> ("error out"=w176:errorcluster, "PhoenixMotorControlDevRef"=w175:T10)  [unwired: 7 in]
  n114 = call <vilib>:"CTRE_Phoenix_MotorControl_ConfigSupplyCurrentLimit.vi"("error in (no error)"=w164, "Supply Current Limit Configuration"=w170, "PhoenixMotorControlDevRef"=w165) -> ("error out"=w174:errorcluster, "PhoenixMotorControlDevRef"=w173:T10)  [unwired: 7 in]
  n115 = call <vilib>:"CTRE_Phoenix_MotorControl_ConfigStatorCurrentLimit.vi"("error in (no error)"=w172, "Stator Current Limit Configuration"=w161, "PhoenixMotorControlDevRef"=w171) -> ()  [unwired: 7 in, 2 out]
  n116 = call <vilib>:"CTRE_Phoenix_MotorControl_ConfigStatorCurrentLimit.vi"("error in (no error)"=w174, "Stator Current Limit Configuration"=w161, "PhoenixMotorControlDevRef"=w173) -> ()  [unwired: 7 in, 2 out]
  n117 = call <vilib>:"CTRE_Phoenix_MotorControl_ConfigStatorCurrentLimit.vi"("error in (no error)"=w178, "Stator Current Limit Configuration"=w161, "PhoenixMotorControlDevRef"=w177) -> ()  [unwired: 7 in, 2 out]
  n118 = call <vilib>:"CTRE_Phoenix_MotorControl_ConfigStatorCurrentLimit.vi"("error in (no error)"=w176, "Stator Current Limit Configuration"=w161, "PhoenixMotorControlDevRef"=w175) -> ()  [unwired: 7 in, 2 out]
  "error out" <- "error in"
